vi "Tester.vi"() -> ()   [LabVIEW 2019, in "TimingDRV Engine.lvlib"]
uses:
  TimingDRV Engine.lvlib
  Processes/Ouput Process/Output Process.lvclass
  C:/Users/XEnderMD/Desktop/CD Project Tools/Source/Engine/Parent Classes/Process/Process.lvclass
  Processes/Input Process/Input Process.lvclass
  Assembler/TypeDefs/Assembler Configuration.ctl
  Assembler/TypeDefs/Process Configuration.ctl
  Parent Classes/Process/Process.lvclass
  <vilib>/NI VeriStand/Custom Device API/Custom Device Engine Event Ref.ctl
  <vilib>/NI VeriStand/Custom Device API/Message (Byte Array).ctl
  <vilib>/NI VeriStand/Custom Device API/Message Response (Byte Array).ctl
  <vilib>/NI VeriStand/Custom Device API/Message (String).ctl
  <vilib>/NI VeriStand/Custom Device API/Message Response (String).ctl
  Assembler/Assembler.lvclass
  <vilib>/NI VeriStand/Custom Device API/Custom Device API.lvlib
panel:
  out "error out":errorcluster
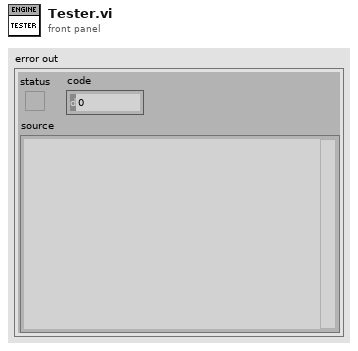
[diagram p1: front panel]
types:
  T1 = typedef "Custom Device API.lvlib/Custom Device Engine Event Ref.ctl" = refnum<event-registration>
  T2 = typedef "TimingDRV Engine.lvlib/Assembler.lvclass/Assembler Configuration.ctl" = cluster{"Process Settings":T3, "Processes":refnum<class "Process.lvclass">[], "CD Engine Event Ref":T1}
  T3 = typedef "TimingDRV Engine.lvlib/Assembler.lvclass/Process Configuration.ctl" = cluster{"Process Timeout":dbl}
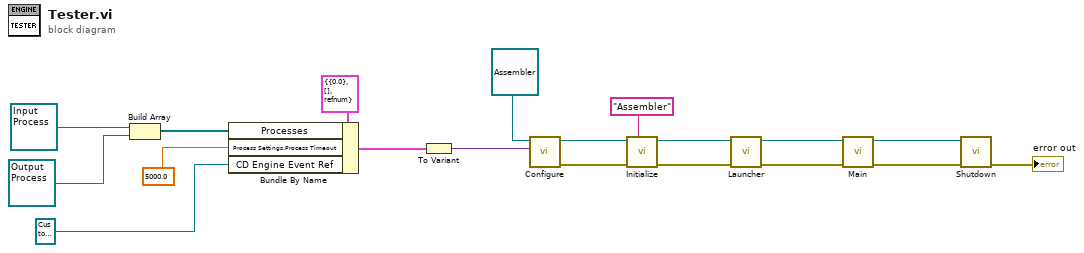
[diagram p0: block diagram]
diagram:
  n1 = Build Array(refnum<class "Input Process.lvclass"> refnum ("TimingDRV Engine.lvlib:Input Process.lvclass"), refnum<class "Output Process.lvclass"> refnum ("TimingDRV Engine.lvlib:Output Process.lvclass")) -> (w16:refnum<class "Process.lvclass">[])
  n2 = Bundle By Name(cluster=T2 {"Process Settings"={"Process Timeout"=0.0}, "Processes"=[], "CD Engine Event Ref"=refnum} ("Assembler Configuration"), "Processes"=w16, "Process Settings.Process Timeout"=5000.0, "CD Engine Event Ref"=T1 refnum) -> (w13:T2)
  n3 = To Variant(anything=w13) -> (Variant=w12:variant)
  n4 = call-dynamic "Configure.vi"("Parameters"=w12, "Assembler in"=refnum<class "Assembler.lvclass"> refnum) -> ("error out"=w11:errorcluster, "Assembler out"=w10:refnum<class "Assembler.lvclass">)  [unwired: 8 in]
  n5 = call-dynamic "Initialize.vi"("Process ID"="Assembler", "error in (no error)"=w11, "Assembler in"=w10) -> ("error out"=w8:errorcluster, "Assembler out"=w7:refnum<class "Assembler.lvclass">)  [unwired: 7 in]
  n6 = call-dynamic "Launcher.vi"("error in (no error)"=w8, "Assembler in"=w7) -> ("error out"=w6:errorcluster, "Assembler out"=w5:refnum<class "Assembler.lvclass">)  [unwired: 8 in]
  n7 = call-dynamic "Main.vi"("error in (no error)"=w6, "Process in"=w5) -> ("error out"=w4:errorcluster, "Process out"=w3:refnum<class "Assembler.lvclass">)  [unwired: 8 in]
  n8 = call-dynamic "Shutdown.vi"("error in (no error)"=w4, "Assembler in"=w3) -> ("error out"=→"error out":errorcluster)  [unwired: 9 in]
